vi "Main.vi"() -> ()   [LabVIEW 2020]
uses:
  <vilib>/nisyscfg/Filter Mode.ctl
  <vilib>/Platform/TimedLoop/XDataNode/timing_clust.ctl
  <vilib>/Platform/TimedLoop/XDataNode/nitl_modes.ctl
  <vilib>/Platform/TimedLoop/XDataNode/wakeup.ctl
  <vilib>/DAQmx/write.llb/DAQmx Write (Digital Bool 1Line 1Point).vi
  <vilib>/DAQmx/read.llb/DAQmx Read (Counter DBL 1Chan 1Samp).vi
  <vilib>/DAQmx/create/channels.llb/DAQmx Create Channel (DO-Digital Output).vi
  <vilib>/DAQmx/miscellaneous.llb/DAQmx Fill In Error Info.vi
  <vilib>/DAQmx/create/channels.llb/DAQmx Create Channel (CI-Position-Linear Encoder).vi
  <vilib>/platform/TimedLoop/XDataNode/XDataNode.xnode
  <vilib>/nisyscfg/nisyscfg.lvlib
  <resource>/objmgr/nisysapi.rc
  <resource>/objmgr/daqmx.rc
  <vilib>/Platform/TimedLoop/XDataNode/XDNodeRunTimeDep.lvlib
panel:
  in  "dt (ms)":i64=10
  out "Current File Size (kB)":dbl
  out "File Location":path
  in  "save":bool
  out "Configuration Complete?":bool
  out "Acquisition Time":timestamp format="%<%H:%M:%S%2u>T"
  out "String Position":dbl(graph)
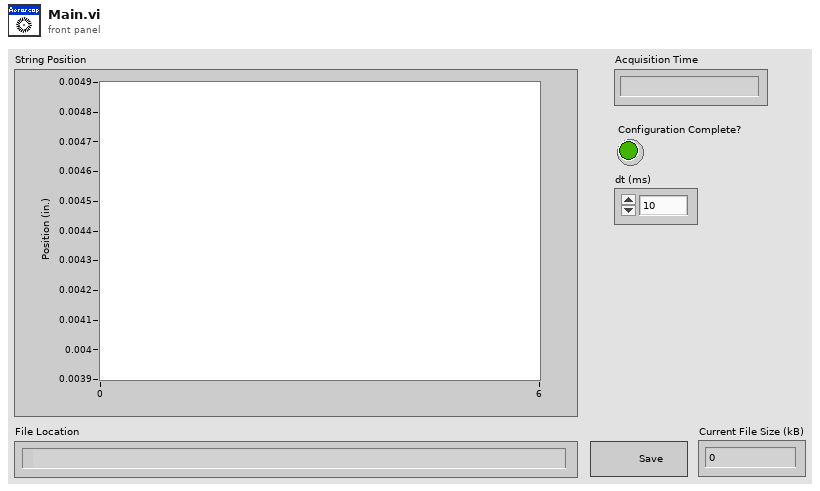
[diagram p1: front panel]
types:
  T1 = typedef "nisyscfg.lvlib/Filter Mode.ctl" = i32
  T2 = cluster{"seconds since 1Jan1904":timestamp, "data":dbl}
  T3 = typedef "XDNodeRunTimeDep.lvlib/timing_clust.ctl" = cluster{"Expected End [f-1]":u64, "Actual End [f-1]":u64, "Finished Late? [f-1]":bool, "Expected End [i-1]":u64, "Actual End [i-1]":u64, "Finished Late? [i-1]":bool, "Expected Start [i]":u64, "Actual Start [i]":u64, "Expected Start [f]":u64, "Actual Start [f]":u64, "Source Name":string, "Structure Name":string, "Period":i64, "Deadline":i64, "Offset":i64, "Start":i64, "Priority":i32, "Timeout":i32, "Mode":T4, "Wakeup Reason":T5, "Error":errorcluster, "Source Type":string, "Secondary Source Type":string, "Global End Time":u64, "Global Start Time":u64, "Frame Duration":u64, "Iteration Duration":u64, "Assigned CPU":i32, "I/O Scan Engine Mode":u32}
  T4 = typedef "XDNodeRunTimeDep.lvlib/nitl_modes.ctl" = enum32{"No Change", "Process missed periods, maintain original phase", "Discard missed periods, maintain original phase", "Process missed periods, ignore original phase", "Discard missed periods, ignore original phase"}
  T5 = typedef "XDNodeRunTimeDep.lvlib/wakeup.ctl" = enum32{"Normal", "Aborted", "Asynchronous wakeup", "Timing source error", "Timed loop error", "Timeout"}
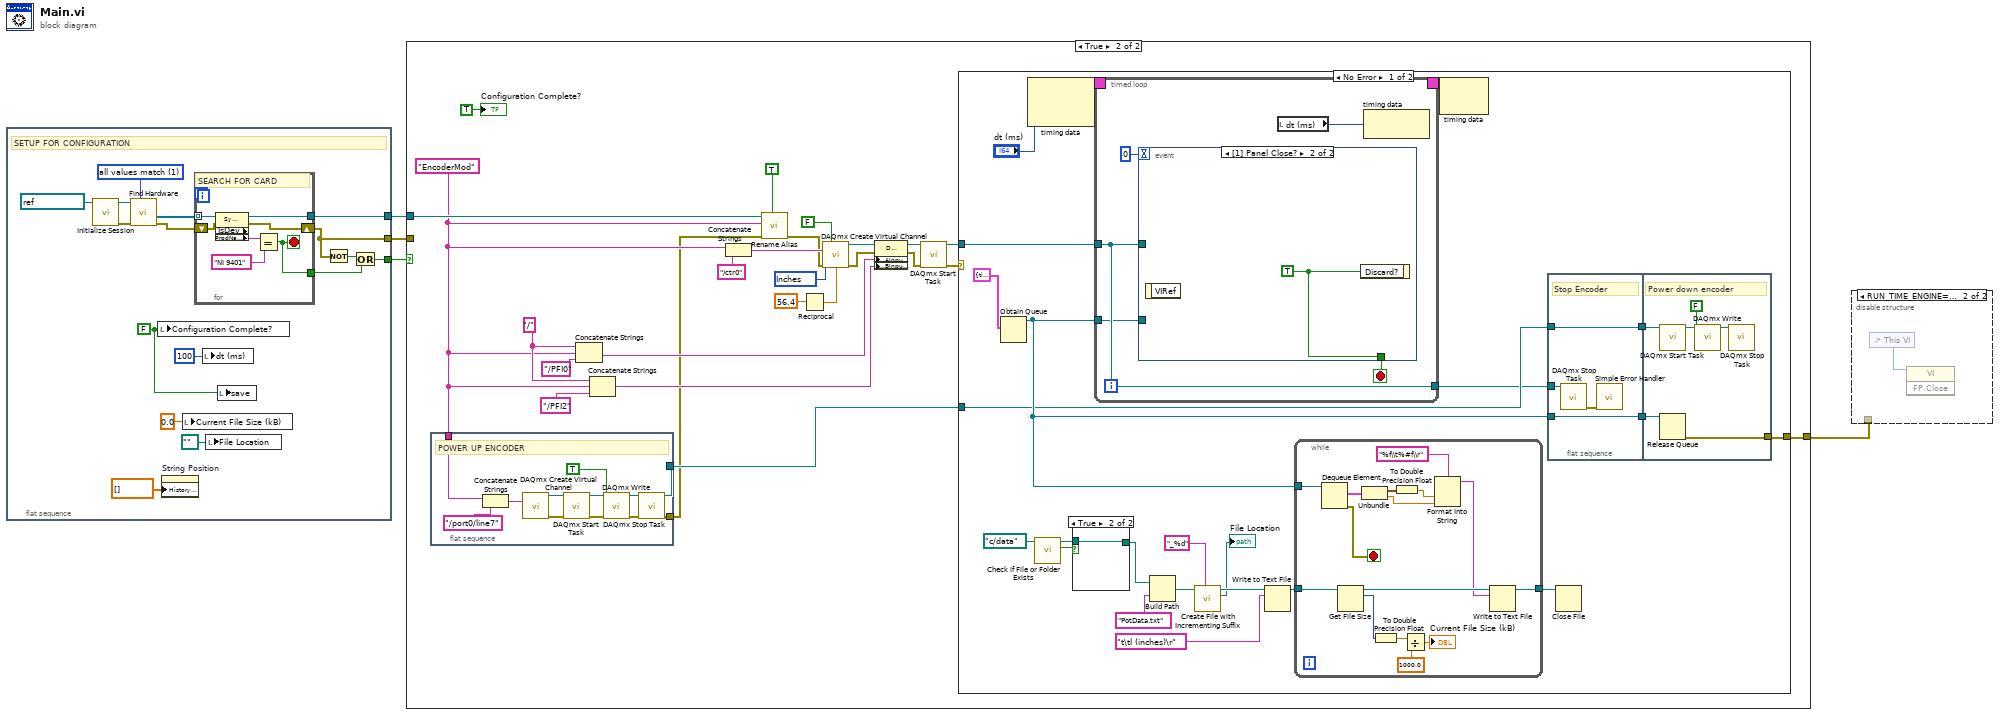
[diagram p0: block diagram]
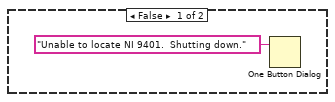
[diagram p3: hidden frame]
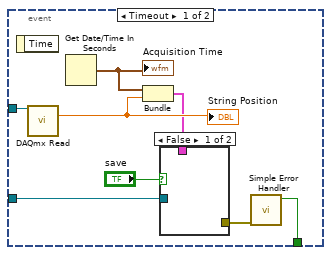
[diagram p4: hidden frame]
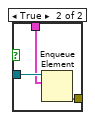
[diagram p5: hidden frame]
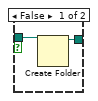
[diagram p6: hidden frame]
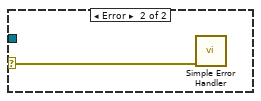
[diagram p7: hidden frame]
diagram:
  n1 = flat-sequence {
    tunnel: [w15] -> w4
    tunnel: [w12] -> w3
    tunnel: [w10] -> w2
    frame #0 {
      w8 = FALSE ("Configuration Complete?")
      w17 = T1 1 items=["all values match"=1, "any value matches"=2, "values do not match"=3, "all properties exist"=4] ("Filter Mode (all values match)")
      # "SETUP FOR CONFIGURATION"
      n2 = call <vilib>:"Initialize Session.vi"("Target (localhost)"=refnum<k21> "localhost") -> ("error out"=w19:errorcluster, "Session out"=w18:refnum<k21>)  [unwired: 9 in]
      n3 = call <vilib>:"Find Hardware.vi"("Filter Mode (all values match)"=w17, "error in (no error)"=w19, "Session in"=w18) -> ("error out"=w14:errorcluster, "Resources out"=w16:refnum<k20>[])  [unwired: 5 in, 2 out]
      n4 = local write "Configuration Complete?"(w8) -> ()
      n5 = property on="String Position" class="WFChart (strict)"("History Data"=dbl[] []) -> ()  [unwired: 2 in, 2 out]
      n6 = local write "Current File Size (kB)"(0.0 ("Current File Size (kB)")) -> ()
      n7 = for {
        tunnel: w16 -> [w27] mode=indexing
        tunnel: [w24] -> w15
        tunnel: [w23] -> w13
        shift-right: [w21] -> w12
        shift-left: w14 -> [w22]
        stop <- w23 stop-if-true
        # "SEARCH FOR CARD"
        n8 = property class="System Hardware" props=["IsDev", "ProdName"](reference=w27, error in=w22) -> (reference out=w24:refnum<k20>, error out=w21:errorcluster, "ProdName"=w26:string)  [unwired: 1 out]
        n9 = Equal?(x=w26, y="NI 9401") -> (x = y?=w23:bool)
      }
      n10 = local write "dt (ms)"(i64 100 ("dt (ms)")) -> ()
      n11 = local write "File Location"(path "" ("File Location")) -> ()
      n12 = local write "save"(w8) -> ()
      n13 = Not(x=w12) -> (.not. x?=w11:bool)
      n14 = Or(x=w11, y=w13) -> (x .or. y?=w10:bool)
    }
  }
  n15 = case shown="True" w2 {
    tunnel: w3 -> [_ _]
    tunnel: w4 -> [_ w52]
    tunnel: [_ w46] -> w1
    frame False {
      n16 = One Button Dialog(message="Unable to locate NI 9401.  Shutting down.") -> ()  [unwired: 1 in, 1 out]
    }
    frame True {
      w33 = "/" ("string")
      w45 = 10379 items=["Meters"=10219, "Inches"=10379, "Ticks"=10304, "From Custom Scale"=10065] ("units")
      w31 = "EncoderMod" ("New Name")
      n17 = flat-sequence {
        tunnel: w31 -> [w64]
        tunnel: [w55] -> w30
        tunnel: [w54] -> w29
        frame #0 {
          # "POWER UP ENCODER"
          n18 = Concatenate Strings(w64, "/port0/line7" ("string")) -> (w63:string)
          n19 = call-poly <vilib>:"DAQmx Create Virtual Channel.vi"("lines"=w63) -> ("task out"=w61:refnum<k21>, "error out"=w60:errorcluster)  [unwired: 13 in]
          n20 = call <vilib>:"DAQmx Start Task.vi"("task/channels in"=w61, "error in"=w60) -> ("task out"=w59:refnum<k21>, "error out"=w58:errorcluster)  [unwired: 12 in]
          n21 = call-poly <vilib>:"DAQmx Write.vi"("task/channels in"=w59, "data"=TRUE, "error in"=w58) -> ("task out"=w57:refnum<k21>, "error out"=w56:errorcluster)  [unwired: 10 in, 1 out]
          n22 = call <vilib>:"DAQmx Stop Task.vi"("task/channels in"=w57, "error in"=w56) -> ("task out"=w55:refnum<k21>, "error out"=w54:errorcluster)  [unwired: 12 in]
        }
      }
      n23 = Concatenate Strings(w33, w31, "/PFI0" ("string")) -> (w39:string)
      n24 = Concatenate Strings(w33, w31, "/PFI2" ("string")) -> (w38:string)
      n25 = Concatenate Strings(w31, "/ctr0" ("string")) -> (w49:string)
      n26 = call <vilib>:"Rename Alias.vi"("Update Dependencies (T)"=TRUE, "error in (no error)"=w29, "New Name"=w31, "Resource in"=w52) -> ("error out"=w34:errorcluster)  [unwired: 4 in, 3 out]
      n27 = Reciprocal(x=56.4 ("distance per pulse")) -> (1/x=w35:dbl)
      n28 = call-poly <vilib>:"DAQmx Create Virtual Channel.vi"("z index enable"=FALSE, "counter"=w49, "units"=w45, "error in"=w34, "distance per pulse"=w35) -> ("task out"=w44:refnum<k21>, "error out"=w42:errorcluster)  [unwired: 9 in]
      n29 = property class="DAQmx Channel"(reference=w44, error in=w42, "CI.Encoder.AInputTerm"=w39, "CI.Encoder.BInputTerm"=w38) -> (reference out=w43:refnum<k21>, error out=w41:errorcluster)
      n30 = call <vilib>:"DAQmx Start Task.vi"("task/channels in"=w43, "error in"=w41) -> ("task out"=w48:refnum<k21>, "error out"=w47:errorcluster)  [unwired: 12 in]
      n31 = case shown="No Error" w47 {
        selector: w47 -> [_ w142]
        tunnel: w48 -> [w88 _]
        tunnel: [w74 _] -> w46
        tunnel: w30 -> [w69 _]
        frame No Error {
          n32 = Obtain Queue(element data type=T2 {"seconds since 1Jan1904"=timestamp(0 s since 1904-01-01), "data"=0.0} ("output cluster")) -> (queue out=w87:refnum<queue>)  [unwired: 4 in, 2 out]
          n33 = node-c288("dt (ms)") -> (w72:T3)  [unwired: 1 in]
          n34 = call <vilib>:"Check if File or Folder Exists.vi"("path"=path "c:/data") -> ("file or folder exists?"=w85:bool, "dup path"=w84:path)  [unwired: 8 in, 1 out]
          n35 = case shown="True" w85 {
            tunnel: w84 -> [w115 w116]
            tunnel: [w114 w116] -> w83
            frame False {
              n36 = Create Folder(path (use dialog)=w115) -> (created path=w114:path)  [unwired: 2 in, 2 out]
            }
            frame True {
            }
          }
          n37 = timed-loop {
            tunnel: w88 -> [w91]
            tunnel: [w91] -> w66
            tunnel: w87 -> [w90]
            timing: w72 -> [_]
            timing-out: [_] -> w71
            stop <- w93 stop-if-true
            n38 = event shown="[1] Panel Close?" {
              selector: _ -> [_ _]
              dyn-events: _ -> [_ _]
              timeout: 0 -> [_ _]
              tunnel: [w104 w108] -> w93
              tunnel: w91 -> [w100 _]
              tunnel: w90 -> [w103 _]
              event Timeout {
                n39 = event-data() -> ()  [unwired: 1 in, 1 out]
                n40 = call-poly <vilib>:"DAQmx Read.vi"("task/channels in"=w100) -> ("data"=w98:dbl)  [unwired: 12 in, 2 out]
                "String Position" <- w98
                n41 = Get Date/Time In Seconds() -> (seconds since 1Jan1904=w99:timestamp)
                "Acquisition Time" <- w99
                n42 = Bundle("seconds since 1Jan1904"=w99, "data"=w98) -> (w97:T2)  [unwired: 1 in]
                n43 = case shown="False" "save" {
                  tunnel: w103 -> [_ w107]
                  tunnel: [_ w106] -> w101
                  tunnel: w97 -> [_ w105]
                  frame False {
                  }
                  frame True {
                    n44 = Enqueue Element(queue=w107, element=w105) -> (error out=w106:errorcluster)  [unwired: 2 in, 2 out]
                  }
                }
                n45 = call <vilib>:"Simple Error Handler.vi"("error in (no error)"=w101) -> ("error?"=w104:bool)  [unwired: 4 in, 4 out]
              }
              event Panel Close? {
                w108 = TRUE
                n46 = event-data() -> ()  [unwired: 1 in, 1 out]
                n47 = event-data("Discard?"=w108) -> ()  [unwired: 1 in, 1 out]
              }
            }
            n48 = local read "dt (ms)"() -> (w89:i64)
            n49 = node-c288(w89) -> ()  [unwired: 1 out]
          }
          n50 = Build Path(base path=w83, name or relative path="PotData.txt") -> (appended path=w76:path)
          n51 = call <vilib>:"Create File with Incrementing Suffix.vi"("format string (\" (%d)\")"="_%d" ("format string (\" (%d)\")"), "file path"=w76) -> ("actual path"=→"File Location":path, "refnum out"=w78:refnum<file>)  [unwired: 7 in, 1 out]
          n52 = Write to Text File(file (use dialog)=w78, text="t\tl (inches)\r") -> (refnum out=w77:refnum<file>)  [unwired: 2 in, 2 out]
          n53 = while {
            tunnel: w87 -> [w141]
            tunnel: w77 -> [w136]
            tunnel: [w139] -> w80
            stop <- w140 stop-if-true
            n54 = Dequeue Element(queue=w141) -> (element=w132:T2, error out=w140:errorcluster)  [unwired: 2 in, 2 out]
            n55 = Get File Size(file=w136) -> (refnum out=w135:refnum<file>, size (in bytes)=w134:i64)  [unwired: 1 in, 1 out]
            n56 = Unbundle(w132) -> ("seconds since 1Jan1904"=w131:timestamp, "data"=w128:dbl)
            n57 = To Double Precision Float(number=w134) -> (double precision float=w133:dbl)
            n58 = To Double Precision Float(number=w131) -> (double precision float=w129:dbl)
            n59 = Divide(x=w133, y=1000.0) -> (x/y=→"Current File Size (kB)":dbl)
            n60 = Format Into String(format string="%f\\t%#f\\r", w129, w128) -> (resulting string=w127:string)  [unwired: 2 in, 1 out]
            n61 = Write to Text File(file (use dialog)=w135, text=w127) -> (refnum out=w139:refnum<file>)  [unwired: 2 in, 2 out]
          }
          n62 = node-c288(w71) -> ()  [unwired: 1 out]
          n63 = flat-sequence {
            tunnel: w69 -> [w119]
            tunnel: w87 -> [w120]
            tunnel: [w120] -> w68
            tunnel: [w119] -> w67
            tunnel: w66 -> [w118]
            tunnel: [w125] -> w74
            tunnel: w68 -> [w126]
            tunnel: w67 -> [w123]
            frame #0 {
              # "Stop Encoder"
              n64 = call <vilib>:"DAQmx Stop Task.vi"("task/channels in"=w118) -> ("error out"=w117:errorcluster)  [unwired: 13 in, 1 out]
              n65 = call <vilib>:"Simple Error Handler.vi"("error in (no error)"=w117) -> ()  [unwired: 4 in, 5 out]
            }
            frame #1 {
              # "Power down encoder"
              n66 = call <vilib>:"DAQmx Start Task.vi"("task/channels in"=w123) -> ("task out"=w122:refnum<k21>)  [unwired: 13 in, 1 out]
              n67 = Release Queue(queue=w126) -> (error out=w125:errorcluster)  [unwired: 2 in, 2 out]
              n68 = call-poly <vilib>:"DAQmx Write.vi"("task/channels in"=w122, "data"=FALSE) -> ("task out"=w121:refnum<k21>)  [unwired: 11 in, 2 out]
              n69 = call <vilib>:"DAQmx Stop Task.vi"("task/channels in"=w121) -> ()  [unwired: 13 in, 2 out]
            }
          }
          n70 = Close File(refnum=w80) -> ()  [unwired: 1 in, 2 out]
        }
        frame Error {
          n71 = call <vilib>:"Simple Error Handler.vi"("error in (no error)"=w142) -> ()  [unwired: 4 in, 5 out]
        }
      }
      "Configuration Complete?" <- TRUE ("Configuration Complete?")
    }
  }
  n72 = disable-structure shown="RUN_TIME_ENGINE==True" {
    disable-tunnel: w1 -> [_ _]
    frame condition #0 (active) {
    }
    frame condition #1 {
      n73 = control-ref of="This VI"() -> (w143:refnum<vi>)
      n74 = invoke class="VI" method="FP.Close"(reference=w143) -> ()  [unwired: 2 in, 3 out]
    }
  }
